vi "table.vi"() -> ()   [LabVIEW 2013]
uses:
  <vilib>/Utility/miscctls.llb/LVRowAndColumnTypeDef.ctl
panel:
  in  "stop":bool
  in  "Table Control":string[][](table)
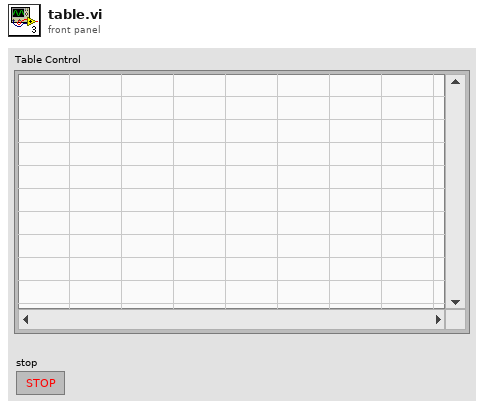
[diagram p1: front panel]
types:
  T1 = typedef "LVRowAndColumnTypeDef.ctl" = cluster{"Row":i32, "Column":i32}
  T2 = enum8{"Enabled", "Disabled", "Disabled and Grayed Out"}
  T3 = typedef "LVPoint32TypeDef.ctl" = cluster{"Horizontal":i32, "Vertical":i32}
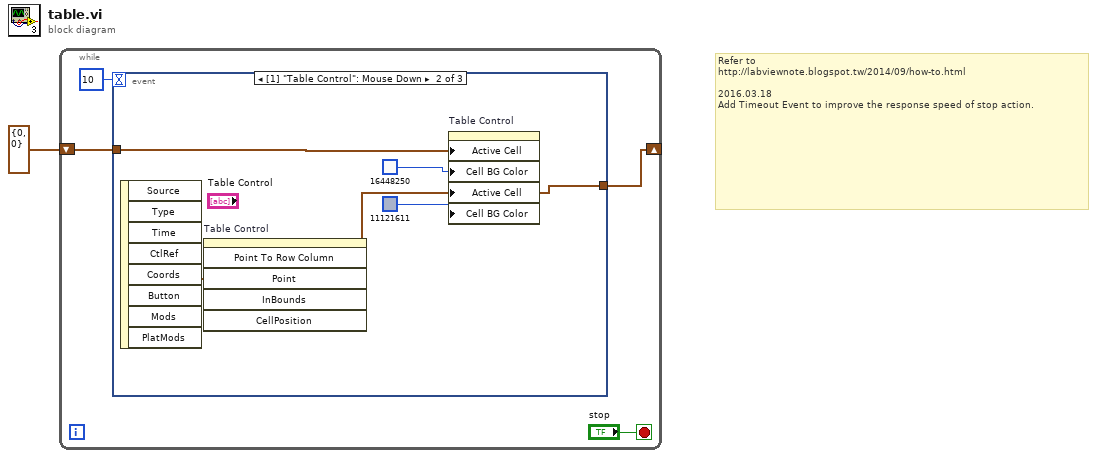
[diagram p0: block diagram]
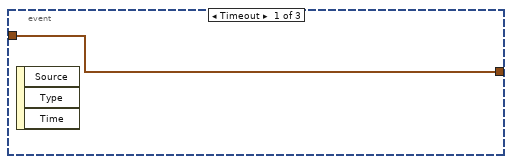
[diagram p2: hidden frame]
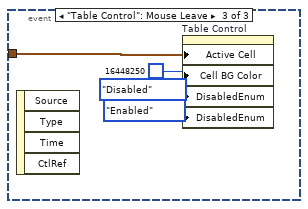
[diagram p3: hidden frame]
diagram:
  # "Refer to \nhttp://labviewnote.blogspot.tw/2014/09/how-to.html\n\n2016.03.18\nAdd Timeout Event to improve the response speed of stop action."
  n1 = while {
    shift-right: [w3] -> _
    shift-left: T1 {"Row"=0, "Column"=0} ("Cell Position") -> [w4]
    stop <- "stop" stop-if-true
    n2 = event shown="[1] \"Table Control\": Mouse Down" {
      selector: _ -> [_ _ _]
      dyn-events: _ -> [_ _ _]
      timeout: 10 -> [_ _ _]
      tunnel: w4 -> [w6 w10 w14]
      tunnel: [w6 w7 _] -> w3
      event Timeout {
        n3 = event-data() -> ()  [unwired: 1 in, 3 out]
      }
      event "Table Control": Mouse Down {
        n4 = event-data() -> ("Coords"=w11:T3)  [unwired: 1 in, 7 out]
        n5 = invoke on="Table Control" class="Tbl (strict)" method="Point To Row Column"("Point"=w11) -> ("CellPosition"=w7:T1)  [unwired: 5 in, 5 out]
        n6 = property on="Table Control" class="Tbl (strict)"("Active Cell"=w10, "Cell BG Color"=u32 16448250 ("Color Box"), "Active Cell"=w7, "Cell BG Color"=u32 11121611 ("Color Box")) -> ()  [unwired: 2 in, 2 out]
      }
      event "Table Control": Mouse Leave {
        n7 = event-data() -> ()  [unwired: 1 in, 4 out]
        n8 = property on="Table Control" class="Tbl (strict)"("Active Cell"=w14, "Cell BG Color"=u32 16448250 ("Color Box"), "DisabledEnum"=T2."Disabled" ("Disabled"), "DisabledEnum"=T2."Enabled" ("Disabled")) -> ()  [unwired: 2 in, 2 out]
      }
    }
  }
